vi "Main.vi"(8 "error in":errorcluster, 11 "_Rescript Msg in":refnum<class "_Msg Rescript.lvclass">) -> (0 "error out":errorcluster, 3 "_Rescript Msg out":refnum<class "_Msg Rescript.lvclass">)   [LabVIEW 2021, in "_Msg Rescript.lvlib" / "_Msg Rescript.lvclass"]
uses:
  _Msg Rescript.lvclass
  _Msg Rescript.lvclass/_Msg Rescript.ctl
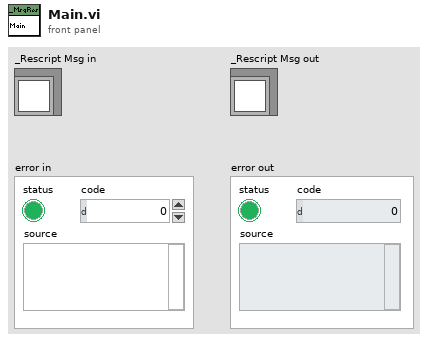
[diagram p1: front panel]
types:
  T1 = typedef "_Msg Rescript.lvlib/_Msg Rescript.lvclass/Ref.ctl" = cluster{"Private Data Control":refnum<vi>, "Private Data Cluster":refnum<vi>, "Msg VI":refnum<vi>, "Init VI":refnum<vi>, "Name VI (Interface)":refnum<vi>, "Name VI":refnum<vi>}
  T2 = map{i32, cluster{"Control":refnum<vi>, "Wire Rule":enum16{"Invalid Wire Rule", "Required", "Recommended", "Optional", "Dynamic Dispatch"}}}
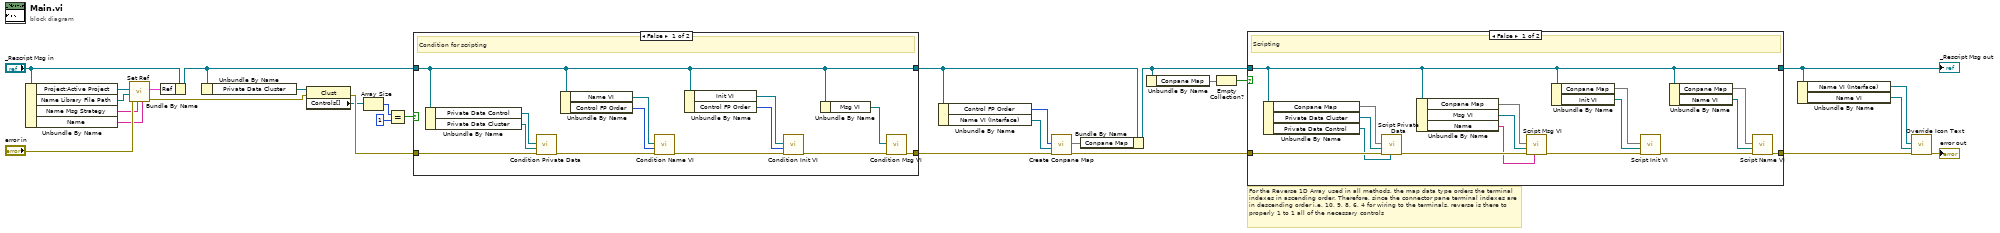
[diagram p0: block diagram]
diagram:
  # "For the Reverse 1D Array used in all methods, the map data type orders the terminal indexes in ascending order. Therefore, since the connector pane terminal indexes are in descending order i.e. 10, 9, 8, 6, 4 for wiring to the terminals, reverse is there to properly 1 to 1 all of the necessary controls"
  n1 = Unbundle By Name("_Rescript Msg in") -> ("Project:Active Project"=w20:refnum<vi>, "Name Library File Path"=w21:path, "Name Msg Strategy"=w22:string, "Name"=w23:string)
  n2 = call "Set Ref.vi"("Name"=w23, "Name Msg Strategy"=w22, "error in"="error in", "Name Library File Path"=w21, "Project:Active Project"=w20) -> ("error out"=w11:errorcluster, "Ref"=w18:T1)  [unwired: 5 in]
  n3 = Bundle By Name(cluster="_Rescript Msg in", "Ref"=w18) -> (w19:refnum<class "_Msg Rescript.lvclass">)
  n4 = Unbundle By Name(w19) -> ("Private Data Cluster"=w12:refnum<vi>)
  n5 = property class="Clust"(reference=w12, error in=w11) -> (error out=w10:errorcluster, "Controls[]"=w3:refnum<vi>[])  [unwired: 1 out]
  n6 = Array Size(array=w3) -> (size(s)=w2:i32)
  n7 = Equal?(x=w2, y=1) -> (x = y?=w4:bool)
  n8 = case shown="False" w4 {
    tunnel: [w42 w44] -> w29
    tunnel: w19 -> [w42 w44]
    tunnel: [w38 w43] -> w15
    tunnel: w10 -> [w39 w43]
    frame False {
      # "Condition for scripting"
      n9 = Unbundle By Name(w42) -> ("Private Data Control"=w41:refnum<vi>, "Private Data Cluster"=w40:refnum<vi>)
      n10 = call "Condition Private Data.vi"("error in"=w39, "Ref.Private Data Cluster"=w40, "Ref.Private Data Control"=w41) -> ("error out"=w32:errorcluster)  [unwired: 8 in]
      n11 = Unbundle By Name(w42) -> ("Name VI"=w30:refnum<vi>, "Control FP Order"=w31:i32[])
      n12 = call "Condition Name VI.vi"("error in"=w32, "Control FP Order"=w31, "Ref.Name VI"=w30) -> ("error out"=w33:errorcluster)  [unwired: 8 in]
      n13 = Unbundle By Name(w42) -> ("Init VI"=w36:refnum<vi>, "Control FP Order"=w35:i32[])
      n14 = call "Condition Init VI.vi"("error in"=w33, "Control FP Order"=w35, "Ref.Init VI"=w36) -> ("error out"=w34:errorcluster)  [unwired: 8 in]
      n15 = Unbundle By Name(w42) -> ("Msg VI"=w37:refnum<vi>)
      n16 = call "Condition Msg VI.vi"("error in"=w34, "Ref.Msg VI"=w37) -> ("error out"=w38:errorcluster)  [unwired: 9 in]
    }
    frame True {
      # "Nothing"
    }
  }
  n17 = Unbundle By Name(w29) -> ("Control FP Order"=w17:i32[], "Name VI (Interface)"=w16:refnum<vi>)
  n18 = call "Create Conpane Map.vi"("error in"=w15, "Ref.Name VI (Interface)"=w16, "Control FP Order"=w17) -> ("error out"=w14:errorcluster, "Conpane Map"=w13:T2)  [unwired: 7 in]
  n19 = Bundle By Name(cluster=w29, "Conpane Map"=w13) -> (w28:refnum<class "_Msg Rescript.lvclass">)
  n20 = Unbundle By Name(w28) -> ("Conpane Map"=w27:T2)
  n21 = Empty Collection?(1:w27) -> (0:w26:bool)
  n22 = case shown="False" w26 {
    tunnel: [w59 w62] -> w9
    tunnel: w28 -> [w59 w62]
    tunnel: [w46 w61] -> w6
    tunnel: w14 -> [w60 w61]
    frame False {
      # "Scripting"
      n23 = Unbundle By Name(w59) -> ("Conpane Map"=w58:T2, "Private Data Cluster"=w57:refnum<vi>, "Private Data Control"=w56:refnum<vi>)
      n24 = call "Script Private Data.vi"("Ref.Private Data Control"=w56, "error in"=w60, "Ref.Private Data Cluster"=w57, "Conpane Map"=w58) -> ("error out"=w53:errorcluster)  [unwired: 7 in]
      n25 = Unbundle By Name(w59) -> ("Conpane Map"=w55:T2, "Msg VI"=w54:refnum<vi>, "Name"=w45:string)
      n26 = call "Script Msg VI.vi"("Name"=w45, "error in"=w53, "Ref.Msg VI"=w54, "Conpane Map"=w55) -> ("error out"=w50:errorcluster)  [unwired: 7 in]
      n27 = Unbundle By Name(w59) -> ("Conpane Map"=w52:T2, "Init VI"=w51:refnum<vi>)
      n28 = call "Script Init VI.vi"("error in"=w50, "Ref.Init VI"=w51, "Conpane Map"=w52) -> ("error out"=w47:errorcluster)  [unwired: 8 in]
      n29 = Unbundle By Name(w59) -> ("Conpane Map"=w49:T2, "Name VI"=w48:refnum<vi>)
      n30 = call "Script Name VI.vi"("error in"=w47, "Ref.Name VI"=w48, "Conpane Map"=w49) -> ("error out"=w46:errorcluster)  [unwired: 8 in]
    }
    frame True {
      # "Nothing"
    }
  }
  "_Rescript Msg out" <- w9
  n31 = Unbundle By Name(w9) -> ("Name VI (Interface)"=w8:refnum<vi>, "Name VI"=w7:refnum<vi>)
  n32 = call "Override Icon Text.vi"("error in"=w6, "Ref.Name VI"=w7, "Ref.Name VI (Interface)"=w8) -> ("error out"=→"error out":errorcluster)  [unwired: 8 in]
